vi "CloseRefDVR.vi"(8 "error in (no error)":errorcluster, 11 "data value reference in":refnum<data-value>) -> (0 "error out":errorcluster, 3 "data value reference out":refnum<data-value>)   [LabVIEW 2023, in "Arithmetic.lvclass"]
doc: "Gets the data value reference of the respective class and closes the subpanel reference"
uses:
  Arithmetic.lvclass
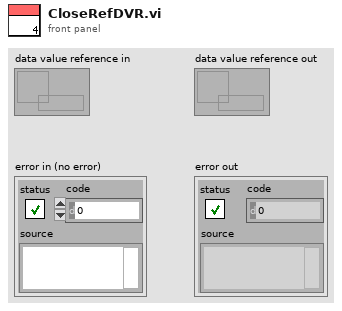
[diagram p1: front panel]
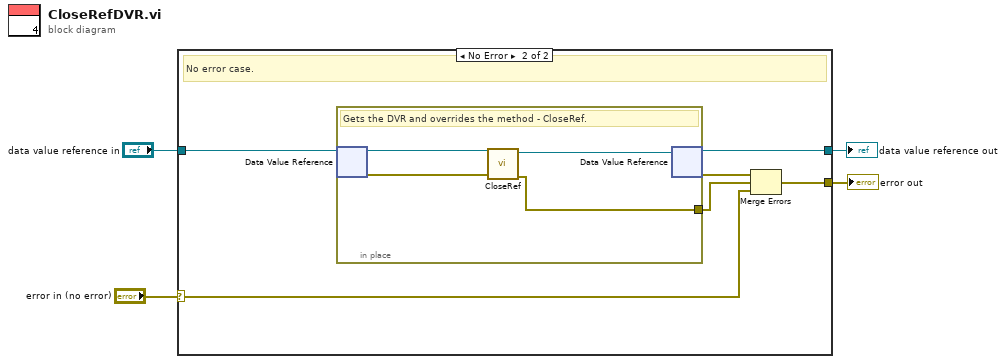
[diagram p0: block diagram]
diagram:
  n1 = case shown="No Error" "error in (no error)" {
    selector: "error in (no error)" -> [w6 w8]
    tunnel: [w6 w7] -> w3
    tunnel: "data value reference in" -> [w5 w12]
    tunnel: [w5 w11] -> w1
    frame Error {
      # "Wire the error cluster across even in the \"No Error\"\ncase so that warnings get propagated."
      # "Error Case."
    }
    frame No Error {
      # "No error case."
      n2 = in-place {
        in-place-border: [w13] -> w9
        # "Gets the DVR and overrides the method - CloseRef."
        n3 = in-place-dvr #1(w12) -> (w16:refnum<class "Arithmetic.lvclass">, w15:errorcluster)
        n4 = call-dynamic "CloseRef.vi"("error in (no error)"=w15, "Arithmetic in"=w16) -> ("error out"=w13:errorcluster, "Arithmetic out"=w14:refnum<class "Arithmetic.lvclass">)  [unwired: 8 in]
        n5 = in-place-dvr #1(w14) -> (w11:refnum<data-value>, w10:errorcluster)
      }
      n6 = Merge Errors(w10, w9, w8) -> (w7:errorcluster)
    }
  }
  "error out" <- w3
  "data value reference out" <- w1
